vi "CAN Working Code.vi"(9 "Stop":bool, 10 "G(T) SK&VW(F)":bool) -> (2 "Fail":bool)   [LabVIEW 2015]
uses:
  Galobal variable_TI.vi
  Project Setup/Globle Variable/GR_Servo.vi
panel:
  in  "CAM_left NG":bool=TRUE
  in  "CAM_left ok":bool=TRUE
  out "string":string
  in  "Start":bool
  in  "Select Model":enum32{"Medium", "Global"}(radio)
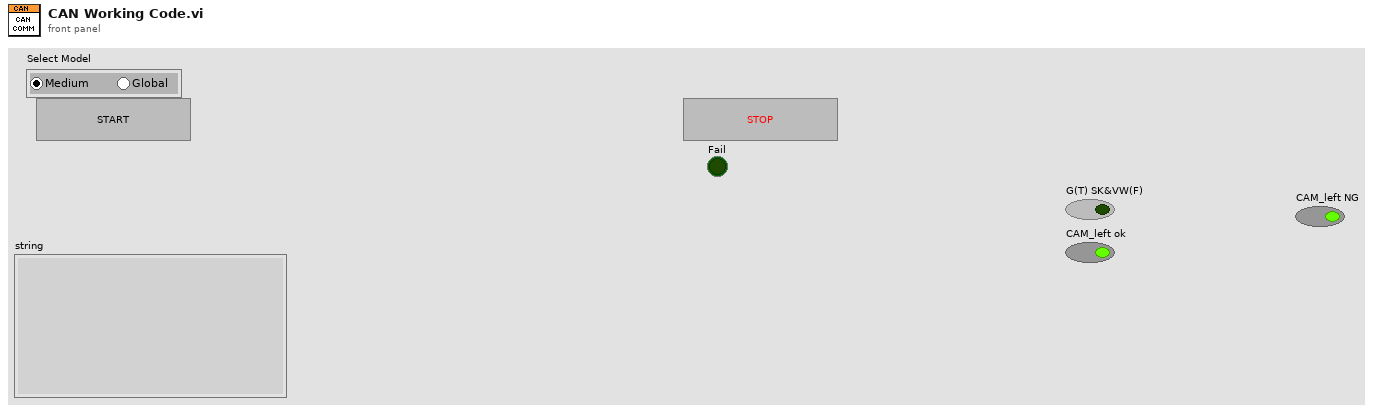
[diagram p1: front panel]
types:
  T1 = typedef "Test Control.ctl" = cluster{"PASS/FAIL Flag":bool, "Numeric Measurement":dbl, "String Measurement":string, "Report Text":string}
  T2 = cluster{"Left CAM OK":bool, "Left CAM NG":bool, "Right CAM OK":bool, "Right CAM NG":bool, "LCD  CAM OK":bool, "LCD CAM NG ":bool}
  T3 = cluster{"Start":bool, "Emergency ":bool, "Reset":bool, "Home":bool, "Safety":bool}
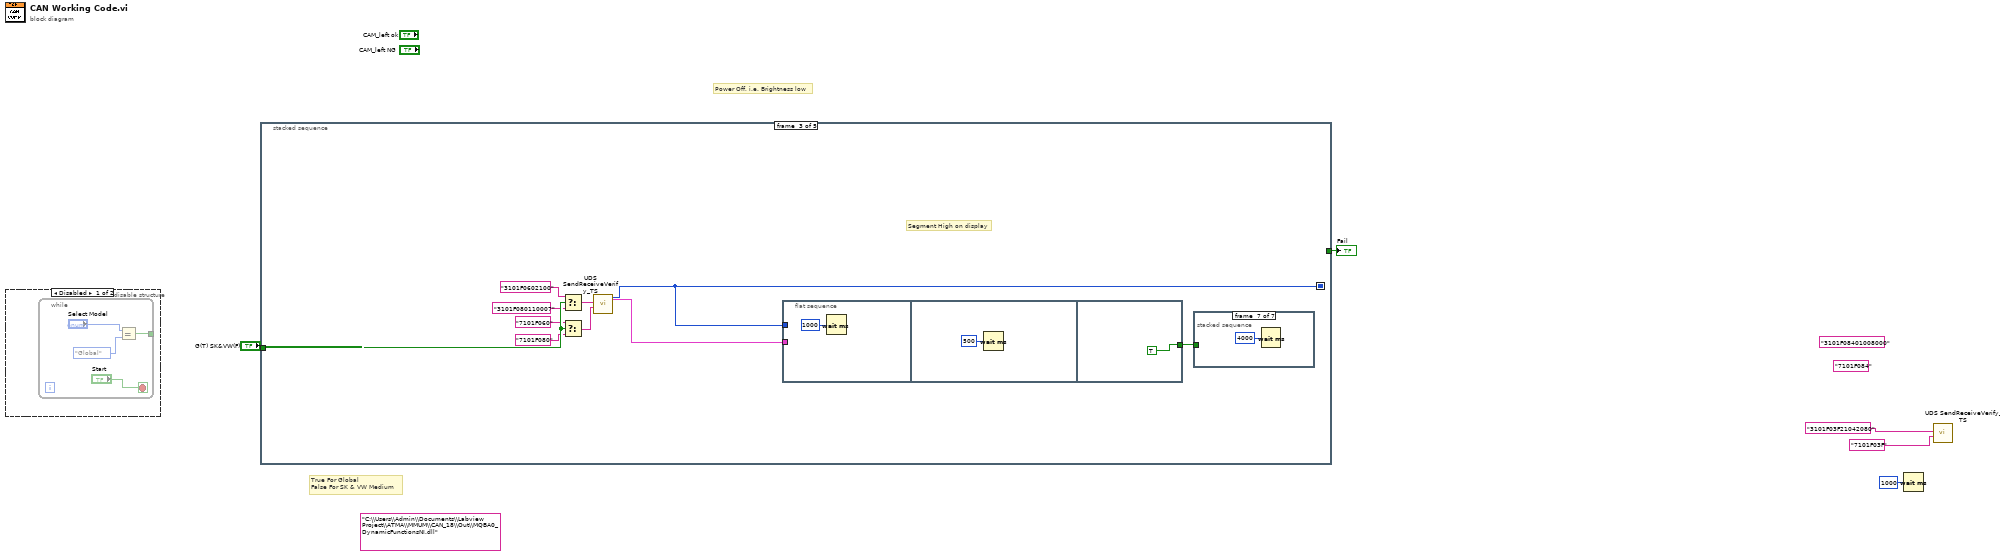
[diagram p0: block diagram]
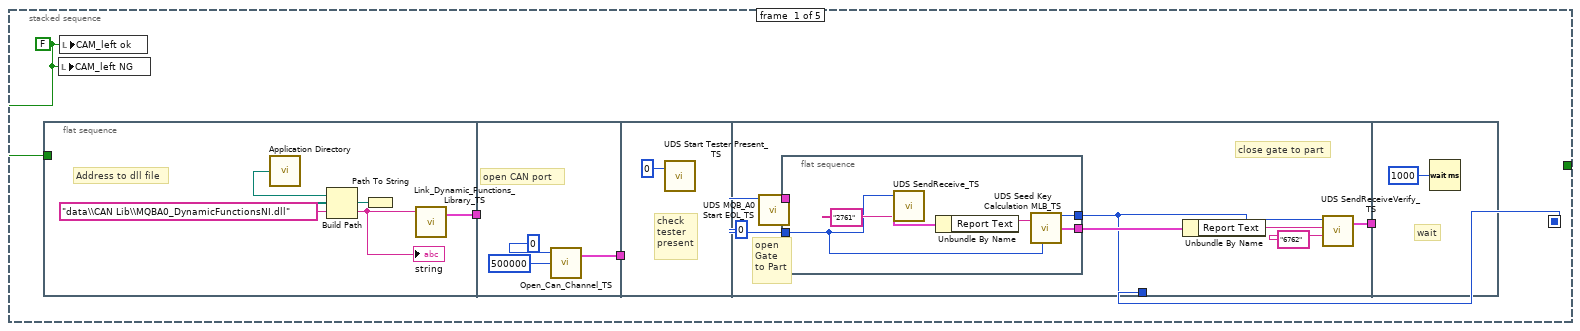
[diagram p3: hidden frame]
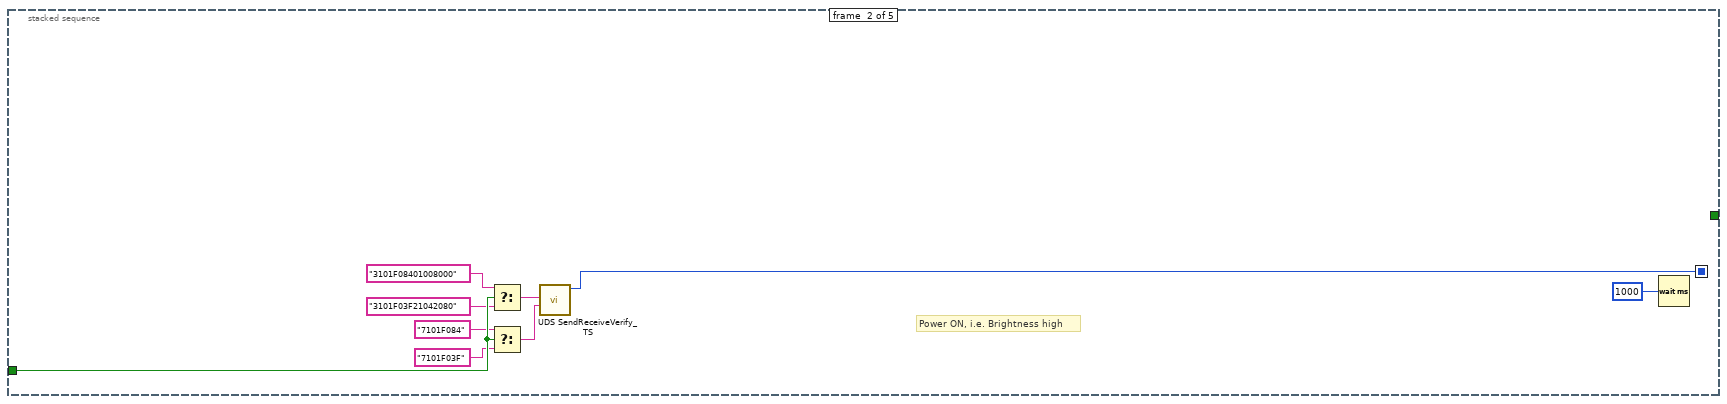
[diagram p4: hidden frame]
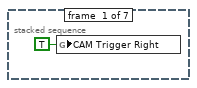
[diagram p5: hidden frame]
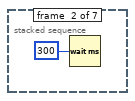
[diagram p6: hidden frame]
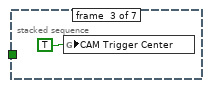
[diagram p7: hidden frame]
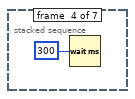
[diagram p8: hidden frame]
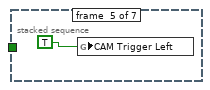
[diagram p9: hidden frame]
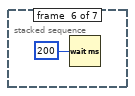
[diagram p10: hidden frame]
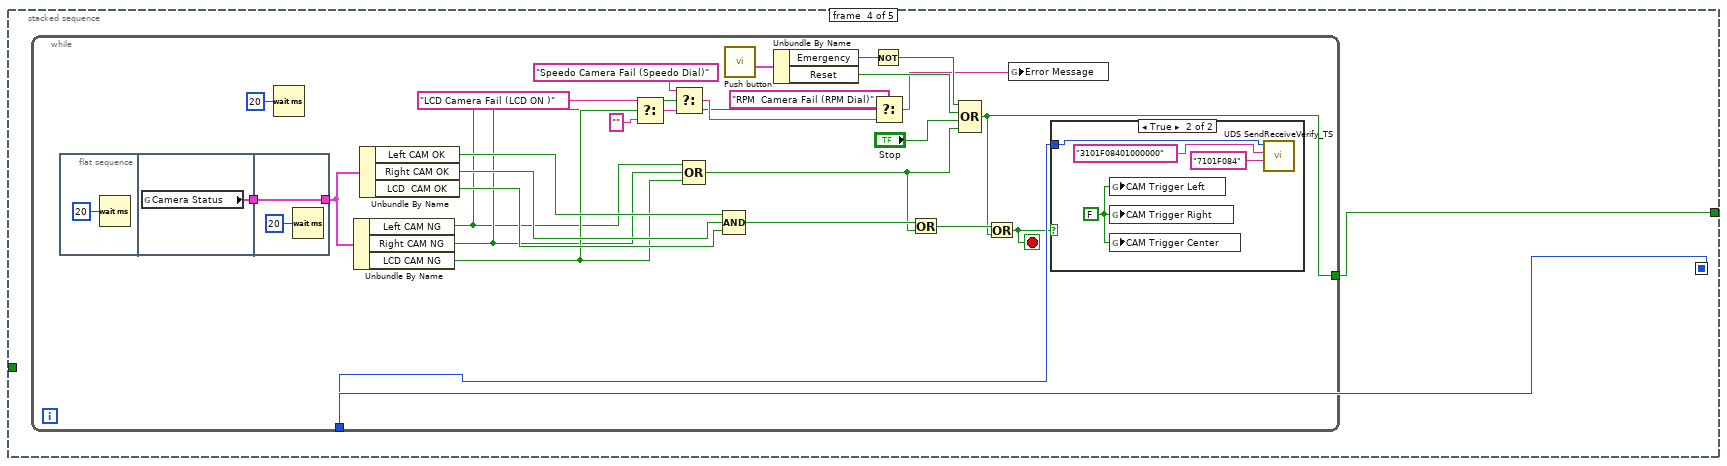
[diagram p11: hidden frame]
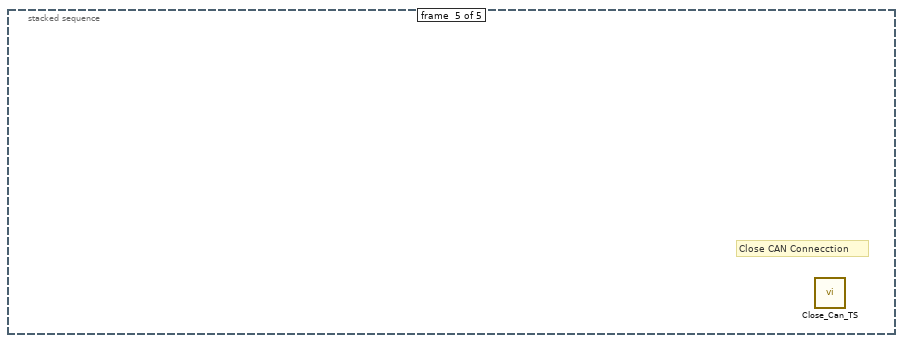
[diagram p13: hidden frame]
diagram:
  (unwired) "C:\\Users\\Admin\\Documents\\Labview Project\\ATMA\\MMUM\\CAN_18\\Out\\MQBA0_DynamicFunctionsNI.dll" ("PathNameDll")
  (unwired) "7101F084" ("expected received data")
  (unwired) "3101F08401008000" ("send data")
  # "Power Off, i.e. Brightness low"
  # "True For Global \nFalse For SK & VW Medium"
  n1 = disable-structure shown="Disabled" {
    frame Disabled {
      n2 = while {
        tunnel: [w7] -> _
        stop <- "Start" stop-if-true
        n3 = Equal?(x="Select Model", y=enum32{"Medium", "Global"}."Global" ("Select Model")) -> (x = y?=w7:bool)
      }
    }
    frame Enabled {
    }
  }
  n4 = stacked-sequence {
    seq-local: [w11 _ _ _ _] -> [_ w44 w48 w67 _]
    tunnel: "G(T) SK&VW(F)" -> [_ w43 w55 _ _]
    tunnel: [_ _ _ w66 _] -> w1
    frame #0 {
      w10 = FALSE ("CAM_left ok")
      n5 = flat-sequence {
        tunnel: [w19] -> w14
        tunnel: w10 -> [_]
        tunnel: w14 -> [_]
        tunnel: [w20] -> w13
        tunnel: w13 -> [_]
        tunnel: [w25] -> w12
        tunnel: [w24] -> w11
        tunnel: w12 -> [_]
        frame #0 {
          # "Address to dll file"
          n6 = call <vilib>:"Application Directory.vi"() -> ("Application Directory"=w16:path)
          n7 = Build Path(base path=w16, name or relative path="data\\CAN Lib\\MQBA0_DynamicFunctionsNI.dll") -> (appended path=w18:path)
          n8 = Path To String(path=w18) -> (string=w15:string)
          "string" <- w15
          n9 = call "Link_Dynamic_Functions_Library_TS.vi"("PathNameDll"=w15) -> ("Test Data"=w19:T1)  [unwired: 3 in]
        }
        frame #1 {
          # "open CAN port"
          n10 = call "Open_Can_Channel_TS.vi"("speed"=u32 500000, "channel"=0) -> ("Test Data"=w20:T1)  [unwired: 2 in]
        }
        frame #2 {
          # "check\ntester\npresent"
          n11 = call "UDS Start Tester Present_TS.vi"("channel"=0) -> ()  [unwired: 2 in, 1 out]
        }
        frame #3 {
          w27 = 0 ("channel")
          # "close gate to part"
          # "open\nGate\nto Part"
          n12 = call "UDS MQB_A0 Start EOL_TS.vi"("channel"=w27) -> ("Test Data"=w30:T1)  [unwired: 10 in]
          n13 = flat-sequence {
            tunnel: [w35] -> w29
            tunnel: w27 -> [w31]
            tunnel: w30 -> [_]
            tunnel: [w31] -> w24
            frame #0 {
              n14 = call "UDS SendReceive_TS.vi"("send data"="2761", "channel"=w31) -> ("Test Data"=w33:T1)  [unwired: 1 in, 2 out]
              n15 = Unbundle By Name(w33) -> ("Report Text"=w34:string)
              n16 = call "UDS Seed Key Calculation MLB_TS.vi"("Seed"=w34) -> ("Test Data"=w35:T1)  [unwired: 1 in]
            }
          }
          n17 = Unbundle By Name(w29) -> ("Report Text"=w28:string)
          n18 = call "UDS SendReceiveVerify_TS.vi"("expected received data"="6762", "send data"=w28, "channel"=w24) -> ("Test Data"=w25:T1)  [unwired: 2 in]
        }
        frame #4 {
          # "wait"
          n19 = Wait (ms)(milliseconds to wait=u32 1000) -> ()  [unwired: 1 out]
        }
      }
      n20 = local write "CAM_left NG"(w10) -> ()
      n21 = local write "CAM_left ok"(w10) -> ()
    }
    frame #1 {
      # "Power ON, i.e. Brightness high"
      n22 = Select(t="3101F08401008000" ("send data"), s=w43, f="3101F03F21042080" ("send data")) -> (s? t:f=w38:string)
      n23 = Select(t="7101F084" ("expected received data"), s=w43, f="7101F03F" ("expected received data")) -> (s? t:f=w37:string)
      n24 = call "UDS SendReceiveVerify_TS.vi"("expected received data"=w37, "send data"=w38, "channel"=w44) -> ()  [unwired: 2 in, 1 out]
      n25 = Wait (ms)(milliseconds to wait=u32 1000) -> ()  [unwired: 1 out]
    }
    frame #2 {
      # "Segment High on display"
      n26 = Select(t="3101F0602100" ("send data"), s=w55, f="3101F080110007" ("send data")) -> (s? t:f=w49:string)
      n27 = Select(t="7101F060" ("expected received data"), s=w55, f="7101F080" ("expected received data")) -> (s? t:f=w50:string)
      n28 = call "UDS SendReceiveVerify_TS.vi"("expected received data"=w50, "send data"=w49, "channel"=w48) -> ("Test Data"=w47:T1)  [unwired: 2 in]
      n29 = flat-sequence {
        tunnel: w48 -> [_]
        tunnel: w47 -> [_]
        tunnel: [TRUE] -> w46
        frame #0 {
          n30 = Wait (ms)(milliseconds to wait=u32 1000) -> ()  [unwired: 1 out]
        }
        frame #1 {
          n31 = Wait (ms)(milliseconds to wait=u32 500) -> ()  [unwired: 1 out]
        }
        frame #2 {
        }
      }
      n32 = stacked-sequence {
        tunnel: w46 -> [_ _ _ _ _ _ _]
        frame #0 {
          n33 = global write "Galobal variable_TI.vi" "CAM Trigger Right"(TRUE ("CAM Trigger Left")) -> ()
        }
        frame #1 {
          n34 = Wait (ms)(milliseconds to wait=u32 300) -> ()  [unwired: 1 out]
        }
        frame #2 {
          n35 = global write "Galobal variable_TI.vi" "CAM Trigger Center"(TRUE ("CAM Trigger Right")) -> ()
        }
        frame #3 {
          n36 = Wait (ms)(milliseconds to wait=u32 300) -> ()  [unwired: 1 out]
        }
        frame #4 {
          n37 = global write "Galobal variable_TI.vi" "CAM Trigger Left"(TRUE ("CAM Trigger Center")) -> ()
        }
        frame #5 {
          n38 = Wait (ms)(milliseconds to wait=u32 200) -> ()  [unwired: 1 out]
        }
        frame #6 {
          n39 = Wait (ms)(milliseconds to wait=u32 4000) -> ()  [unwired: 1 out]
        }
      }
    }
    frame #3 {
      n40 = while {
        tunnel: w67 -> [w94]
        tunnel: [w85] -> w66
        stop <- w92 stop-if-true
        n41 = flat-sequence {
          tunnel: [w96] -> w68
          tunnel: [w98] -> w75
          tunnel: w68 -> [w98]
          frame #0 {
            n42 = Wait (ms)(milliseconds to wait=u32 20) -> ()  [unwired: 1 out]
          }
          frame #1 {
            n43 = global read "Galobal variable_TI.vi" "Camera Status"() -> (w96:T2)
          }
          frame #2 {
            n44 = Wait (ms)(milliseconds to wait=u32 20) -> ()  [unwired: 1 out]
          }
        }
        n45 = Wait (ms)(milliseconds to wait=u32 20) -> ()  [unwired: 1 out]
        n46 = Unbundle By Name(w75) -> ("Left CAM NG"=w69:bool, "Right CAM NG"=w70:bool, "LCD CAM NG"=w71:bool)
        n47 = Unbundle By Name(w75) -> ("Left CAM OK"=w74:bool, "Right CAM OK"=w73:bool, "LCD  CAM OK"=w72:bool)
        n48 = Select(t="LCD Camera Fail (LCD ON )", s=w71, f="") -> (s? t:f=w81:string)
        n49 = Select(t="Speedo Camera Fail (Speedo Dial)", s=w70, f=w81) -> (s? t:f=w79:string)
        n50 = Compound Arithmetic op=OR(w69, w70, w71) -> (w78:bool)
        n51 = Compound Arithmetic op=AND(w74, w73, w72) -> (w86:bool)
        n52 = call "Push button.vi"() -> ("Push Button"=w91:T3)  [unwired: 9 in, 2 out]
        n53 = Unbundle By Name(w91) -> ("Emergency"=w90:bool, "Reset"=w88:bool)
        n54 = Not(x=w90) -> (.not. x?=w89:bool)
        n55 = Select(t="RPM  Camera Fail (RPM Dial)", s=w69, f=w79) -> (s? t:f=w76:string)
        n56 = Or(x=w86, y=w78) -> (x .or. y?=w93:bool)
        n57 = Compound Arithmetic op=OR(w89, w88, "Stop", w78) -> (w85:bool)
        n58 = Or(x=w93, y=w85) -> (x .or. y?=w92:bool)
        n59 = global write "GR_Servo.vi" "Error Message"(w76) -> ()
        n60 = case shown="True" w92 {
          tunnel: w94 -> [_ w100]
          frame False {
          }
          frame True {
            w99 = FALSE ("CAM Trigger Right")
            n61 = global write "Galobal variable_TI.vi" "CAM Trigger Left"(w99) -> ()
            n62 = global write "Galobal variable_TI.vi" "CAM Trigger Right"(w99) -> ()
            n63 = global write "Galobal variable_TI.vi" "CAM Trigger Center"(w99) -> ()
            n64 = call "UDS SendReceiveVerify_TS.vi"("expected received data"="7101F084", "send data"="3101F08401000000", "channel"=w100) -> ()  [unwired: 2 in, 1 out]
          }
        }
      }
    }
    frame #4 {
      # "Close CAN Connecction"
      n65 = call "Close_Can_TS.vi"() -> ()  [unwired: 3 in, 1 out]
    }
  }
  "Fail" <- w1
  n66 = Wait (ms)(milliseconds to wait=u32 1000) -> ()  [unwired: 1 out]
  n67 = call "UDS SendReceiveVerify_TS.vi"("expected received data"="7101F03F", "send data"="3101F03F21042080") -> ()  [unwired: 3 in, 1 out]
